vi "ui_DataLog Query Database.vi"(0 "prompt":string) -> (4 "OK?":bool, 8 "database":string)   [LabVIEW 2012]
doc: "Shows a convenient dialog for selecting a database."
uses:
  served/DataLog Databases_srv.ctl
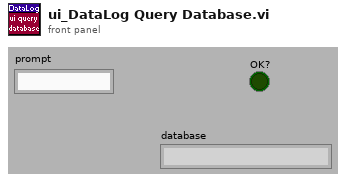
[diagram p1: front panel]
types:
  T1 = typedef "DataLog Databases_srv.ctl" = refnum<vi>
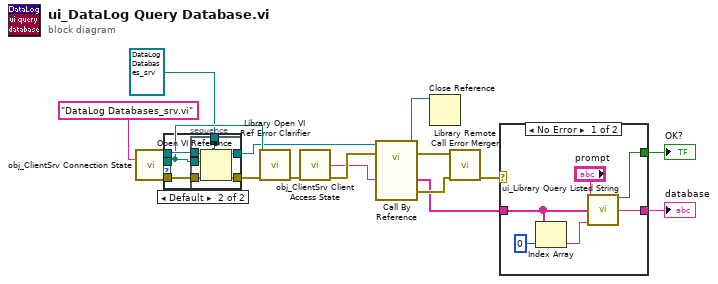
[diagram p0: block diagram]
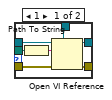
[diagram p2: hidden frame]
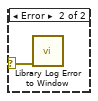
[diagram p3: hidden frame]
diagram:
  n1 = call "obj_ClientSrv Connection State.vi"("machine{connect}/VI{get state} name (local/no path resolution)"="DataLog Databases_srv.vi") -> ("server app ref"=w5:refnum<vi>, "resolved server path"=w4:path, "error out"=w3:errorcluster)  [unwired: 7 in, 5 out]
  n2 = stacked-sequence {
    tunnel: [w23] -> w2
    tunnel: [w22] -> w6
    tunnel: w3 -> [w21]
    tunnel: w5 -> [w20]
    tunnel: w4 -> [w19]
    tunnel: T1 refnum ("databases") -> [w18]
    frame #0 {
      # "avoid LV8 complaints"
      n3 = Path to Array of Strings(0:w19) -> (2:w24:string[])  [unwired: 1 out]
      n4 = Array Size(array=w24) -> (size(s)=w25:i32)
      n5 = case shown="Default" w25 {
        tunnel: w19 -> [w32 w38]
        tunnel: w20 -> [w30 w37]
        tunnel: [w28 w33] -> w23
        tunnel: [w26 w36] -> w22
        tunnel: w18 -> [w27 w35]
        tunnel: w21 -> [w29 w34]
        frame 1 {
          n6 = Path To String(path=w32) -> (string=w31:string)
          n7 = Open VI Reference(type specifier VI Refnum (for type only)=w27, application reference (local)=w30, vi path=w31, error in (no error)=w29) -> (vi reference=w28:T1, error out=w26:errorcluster)  [unwired: 2 in]
        }
        frame Default {
          n8 = Open VI Reference(type specifier VI Refnum (for type only)=w35, application reference (local)=w37, vi path=w38, error in (no error)=w34) -> (vi reference=w33:T1, error out=w36:errorcluster)  [unwired: 2 in]
        }
      }
    }
  }
  n9 = call "Library Open VI Ref Error Clarifier.vi"("VI path"=w4, "called VI error (no error)"=w6) -> ("error out"=w14:errorcluster)  [unwired: 13 in]
  n10 = call "obj_ClientSrv Client Access State.vi"("error in (no error)"=w14) -> ("certificate"=w9:string, "error out"=w17:errorcluster)  [unwired: 13 in]
  n11 = call-by-ref "?"(reference=w2, error in=w17, "certificate in"=w9) -> (reference out=w11:T1, error out=w15:errorcluster, "database names"=w8:string[], 15:"error out"=w16:errorcluster)  [unwired: 13 in]
  n12 = Close Reference(reference=w11) -> ()  [unwired: 1 in, 1 out]
  n13 = call "Library Remote Call Error Merger.vi"("call by reference node error"=w15, "called VI error (no error)"=w16) -> ("error out"=w7:errorcluster)  [unwired: 13 in]
  n14 = case shown="No Error" w7 {
    selector: w7 -> [_ w45]
    tunnel: [w44 _] -> w13
    tunnel: w8 -> [w41 _]
    tunnel: [w43 _] -> w12
    frame No Error {
      n15 = Index Array(array=w41, index=0) -> (element=w39:string)
      n16 = call "ui_Library Query Listed String.vi"("prompt"="prompt", "list of strings"=w41, "default (persist)"=w39) -> ("OKed?"=w44:bool, "selected string"=w43:string)  [unwired: 11 in]
    }
    frame Error {
      n17 = call "Library Log Error to Window.vi"("error in (no error)"=w45) -> ()  [unwired: 13 in, 2 out]
    }
  }
  "database" <- w12
  "OK?" <- w13
